vi "N_forsed_bits64.vi"(3 "IN":u64 format="%b") -> (1 "N_forsed_bits":u64)   [LabVIEW 2019, in "Logik.lvlib"]
uses:
  Logik.lvlib
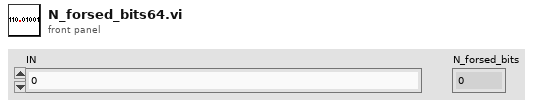
[diagram p1: front panel]
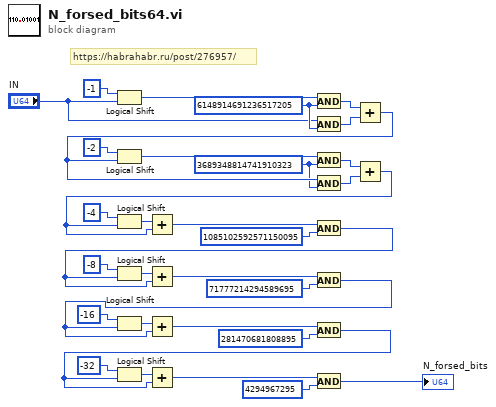
[diagram p0: block diagram]
diagram:
  w11 = u64 3689348814741910323 ("y")
  w8 = u64 6148914691236517205 ("y")
  # "https://habrahabr.ru/post/276957/"
  n1 = Logical Shift(y=i16 -1, x="IN") -> (x << y=w14:u64)
  n2 = And(x=w14, y=w8) -> (x .and. y?=w9:u64)
  n3 = And(x="IN", y=w8) -> (x .and. y?=w10:u64)
  n4 = Add(x=w9, y=w10) -> (x+y=w18:u64)
  n5 = Logical Shift(y=i16 -2, x=w18) -> (x << y=w17:u64)
  n6 = And(x=w17, y=w11) -> (x .and. y?=w12:u64)
  n7 = And(x=w18, y=w11) -> (x .and. y?=w13:u64)
  n8 = Add(x=w12, y=w13) -> (x+y=w21:u64)
  n9 = Logical Shift(y=i16 -4, x=w21) -> (x << y=w20:u64)
  n10 = Add(x=w20, y=w21) -> (x+y=w22:u64)
  n11 = And(x=w22, y=u64 1085102592571150095) -> (x .and. y?=w31:u64)
  n12 = Logical Shift(y=i16 -8, x=w31) -> (x << y=w26:u64)
  n13 = Add(x=w26, y=w31) -> (x+y=w25:u64)
  n14 = And(x=w25, y=u64 71777214294589695) -> (x .and. y?=w32:u64)
  n15 = Logical Shift(y=i16 -16, x=w32) -> (x << y=w28:u64)
  n16 = Add(x=w28, y=w32) -> (x+y=w29:u64)
  n17 = And(x=w29, y=u64 281470681808895) -> (x .and. y?=w3:u64)
  n18 = Logical Shift(y=i16 -32, x=w3) -> (x << y=w6:u64)
  n19 = Add(x=w6, y=w3) -> (x+y=w5:u64)
  n20 = And(x=w5, y=u64 4294967295) -> (x .and. y?=→"N_forsed_bits":u64)
